vi "CSC_XYZ0toGlobal.vi"(6 "Dir(xyz0->global)":enum16{"global->xyz0", "xyz0->global"}(ring)=enum."xyz0->global", 8 "error in (no error)":errorcluster, 9 "Vin":dbl[](array[numeric])=[0.0, 0.0, 0.0], 10 "Pin":dbl[](array[numeric])=[0.0, 0.0, 0.0], 11 "CSC In":refnum<class "CableSerialChain.lvclass">) -> (0 "error out":errorcluster, 1 "Vout":dbl[](array[numeric]), 2 "Pout":dbl[](array[numeric]), 3 "CSC Oout":refnum<class "CableSerialChain.lvclass">)   [LabVIEW 2015, in "CableSerialChain.lvclass"]
uses:
  CableSerialChain.lvclass
  CableSerialChain.lvclass/CableSerialChain.ctl
  <vilib>/Analysis/BLAS.llb/LV_Transpose.ctl
  <vilib>/Analysis/BLAS.llb/dgemv - General Matrix-Vector Product (DBL).vi
  <vilib>/Analysis/NI_AALBLAS.lvlib
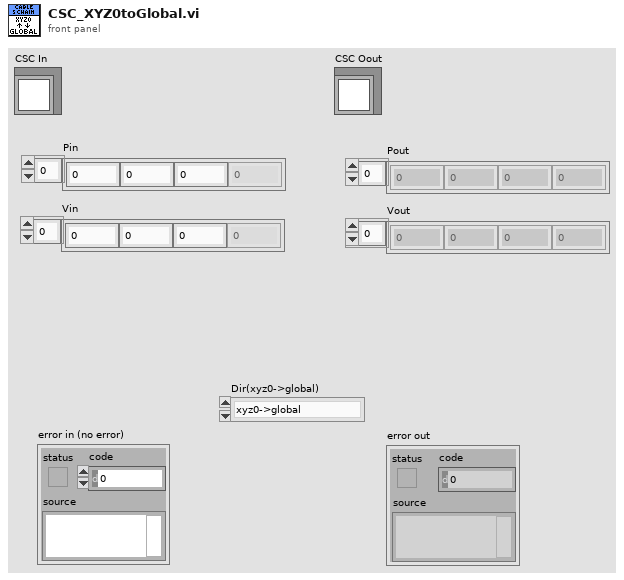
[diagram p1: front panel]
types:
  T1 = typedef "NI_Matrix.lvlib/RealMatrix.ctl" = dbl[][]
  T2 = typedef "NI_AALBLAS.lvlib/LV_Transpose.ctl" = i32
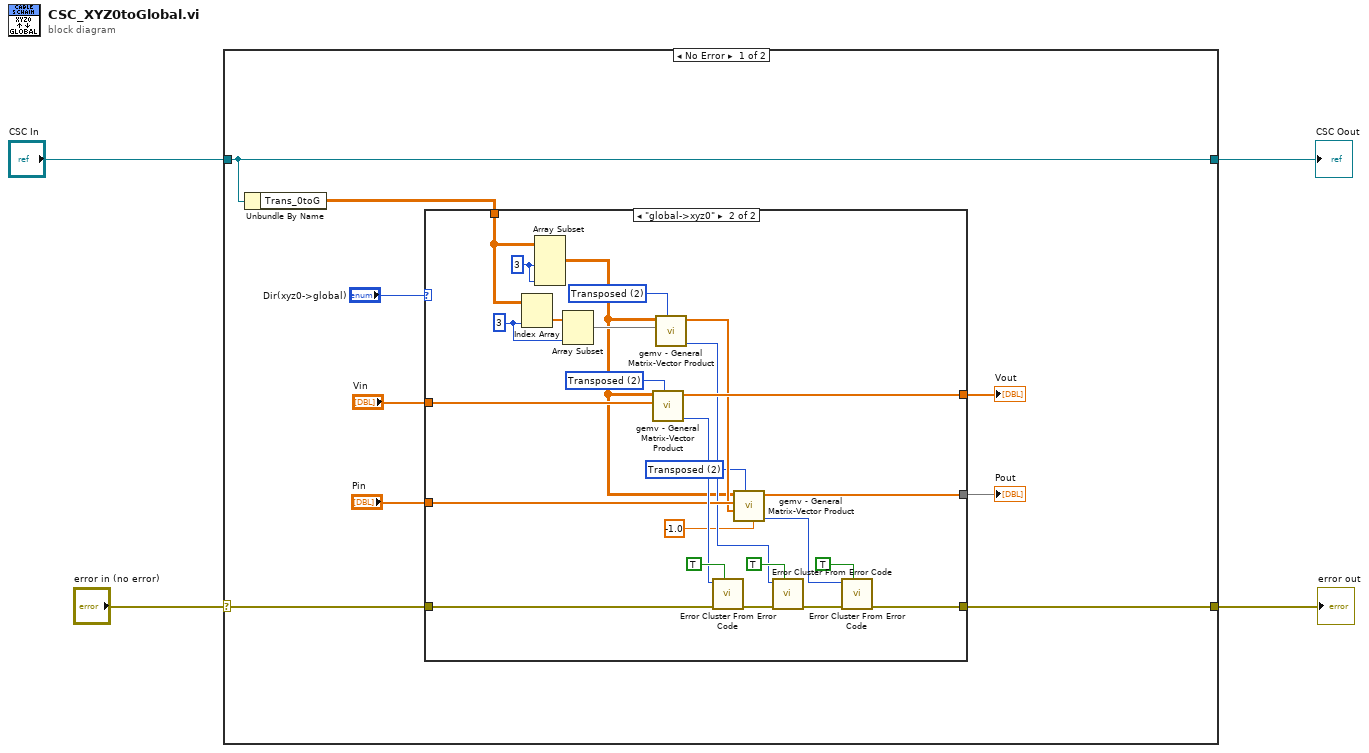
[diagram p0: block diagram]
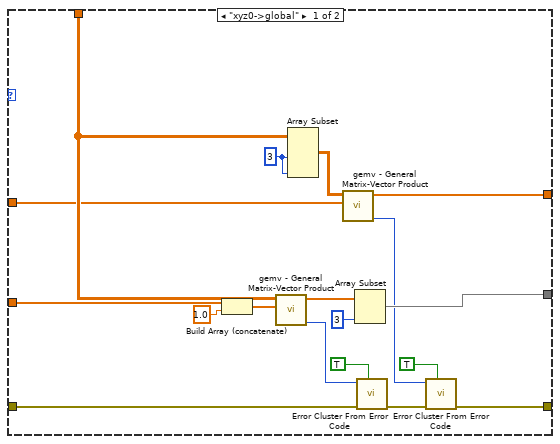
[diagram p2: hidden frame]
diagram:
  n1 = case shown="No Error" "error in (no error)" {
    selector: "error in (no error)" -> [w7 w57]
    tunnel: [w9 w57] -> w4
    tunnel: "CSC In" -> [w5 w58]
    tunnel: [w5 w58] -> w1
    frame No Error {
      n2 = Unbundle By Name(w5) -> ("Trans_0toG"=w6:T1)
      n3 = case shown="\"global->xyz0\"" "Dir(xyz0->global)" {
        tunnel: w7 -> [w31 w44]
        tunnel: "Pin" -> [w30 w41]
        tunnel: [w25 w39] -> w12
        tunnel: w6 -> [w22 w49]
        tunnel: "Vin" -> [w20 w54]
        tunnel: [w18 w53] -> w10
        tunnel: [w15 w51] -> w9
        frame "xyz0->global" {
          w21 = 3
          n4 = Build Array (concatenate)(w30, 1.0) -> (w28:dbl[])
          n5 = call-poly <vilib>:"gemv - General Matrix-Vector Product.vi"("x"=w28, "A"=w22) -> ("error"=w24:i32, "dgemv"=w27:dbl[])  [unwired: 8 in]
          n6 = Array Subset(array=w22, length (row)=w21, length (col)=w21) -> (w19:T1)  [unwired: 2 in]
          n7 = call-poly <vilib>:"gemv - General Matrix-Vector Product.vi"("x"=w20, "A"=w19) -> ("error"=w17:i32, "dgemv"=w18:dbl[])  [unwired: 8 in]
          n8 = Array Subset(array=w27, length=3) -> (w25:dbl[])  [unwired: 1 in]
          n9 = call <vilib>:"Error Cluster From Error Code.vi"("show call chain? (False)"=TRUE, "error in (no error)"=w31, "error code (0)"=w24) -> ("error out"=w16:errorcluster)  [unwired: 6 in]
          n10 = call <vilib>:"Error Cluster From Error Code.vi"("show call chain? (False)"=TRUE, "error in (no error)"=w16, "error code (0)"=w17) -> ("error out"=w15:errorcluster)  [unwired: 6 in]
        }
        frame "global->xyz0" {
          w32 = T2 2 items=["Direct", "Conjugated & Transposed", "Transposed"] ("operation A")
          w33 = T2 2 items=["Direct", "Conjugated & Transposed", "Transposed"] ("operation A")
          w34 = T2 2 items=["Direct", "Conjugated & Transposed", "Transposed"] ("operation A")
          w47 = 3 ("index")
          w55 = 3
          n11 = Index Array(array=w49, index (col)=w47) -> (element=w48:dbl[])  [unwired: 1 in]
          n12 = Array Subset(array=w49, length (row)=w55, length (col)=w55) -> (w35:T1)  [unwired: 2 in]
          n13 = Array Subset(array=w48, length=w47) -> (w46:dbl[])  [unwired: 1 in]
          n14 = call-poly <vilib>:"gemv - General Matrix-Vector Product.vi"("operation A"=w33, "x"=w54, "A"=w35) -> ("error"=w42:i32, "dgemv"=w53:dbl[])  [unwired: 7 in]
          n15 = call-poly <vilib>:"gemv - General Matrix-Vector Product.vi"("operation A"=w34, "x"=w46, "A"=w35) -> ("error"=w38:i32, "dgemv"=w37:dbl[])  [unwired: 7 in]
          n16 = call <vilib>:"Error Cluster From Error Code.vi"("show call chain? (False)"=TRUE, "error in (no error)"=w44, "error code (0)"=w42) -> ("error out"=w43:errorcluster)  [unwired: 6 in]
          n17 = call-poly <vilib>:"gemv - General Matrix-Vector Product.vi"("beta"=-1.0, "operation A"=w32, "y"=w37, "x"=w41, "A"=w35) -> ("error"=w40:i32, "dgemv"=w39:dbl[])  [unwired: 5 in]
          n18 = call <vilib>:"Error Cluster From Error Code.vi"("show call chain? (False)"=TRUE, "error in (no error)"=w43, "error code (0)"=w38) -> ("error out"=w52:errorcluster)  [unwired: 6 in]
          n19 = call <vilib>:"Error Cluster From Error Code.vi"("show call chain? (False)"=TRUE, "error in (no error)"=w52, "error code (0)"=w40) -> ("error out"=w51:errorcluster)  [unwired: 6 in]
        }
      }
      "Pout" <- w12
      "Vout" <- w10
    }
    frame Error {
    }
  }
  "error out" <- w4
  "CSC Oout" <- w1
